vi "SOUR_POW_CORR_COLL_ITER_NTOL.vi"(0 "VISA IN":refnum<visa-resource-name>, 1 "Port number":i32, 2 "Tolerance Value(dBm)":dbl, 5 "error in":errorcluster, 7 "Channel":i32) -> (14 "VISA Out":refnum<visa-resource-name>, 19 "error out":errorcluster)   [LabVIEW 2018, in "PNA-X.lvlib"]
doc: "SOURce:POWer:CORRection:COLLect:ITERation:NTOLerance <num> \n1839\n\n(Read-Write) This command, along with SOUR:POW:CORR:COLL:ITER:COUNT describes the \nnumber of ADUSTMENTS to make to the source power. \nSets the maximum desired deviation from the sum of the test port power and the offset value. Power \nREADINGS (performed by SOUR:POW:CORR:COLL:AVER:COUNT and \nSOUR:POW:CORR:COLL:AVER:NTOLerance) will continue to be made, and source power \nadjusted, until a measurement is within this tolerance value or the max number of measurements has \nbeen met. The last value is the valid measurement for that data point. \nLearn more. \nParameters \n<cnum> Any existing channel number. If unspecified, value is set to 1 \n<port> Port number to correct for source power. If unspecified, value is set to 1. \n<num> Tolerance value in dBm. Choose any number between 0 and 5 \nExamples SOUR:POW:CORR:COLL:ITER:NTOL .005 \nsource:power:correction:collect:iteration:ntolerance .1 \nQuery Syntax SOURce:POWer:CORRection:COLLect:ITERation:NTOLerance? \nReturn Type Numeric \nDefault .05 \nSOURce<cnum>:POWer<port>:CORRection:COLLect:METHod <char> Superseded \nThis command is replaced with SOUR:POW:CORR:COLLect[:ACQuire] which now specifies the \nmethod and the device. \n(Read-Write) Selects the calibration method to be used for the source power cal acquisition. \nParameters \n<cnum> Any existing channel number. If unspecified, value is set to 1 \n<port> Port number to correct for source power. If unspecified, value is set to 1. \n<char> Choose from: \nNONE - No Cal method \nPMETer - Power Meter is used for all readings. (same as \"fast iteration\" box \nnot checked on dialog box) \nPMReceiver - Power meter for the first iteration; then use the reference \nreceiver for remaining readings if necessary (same as \"fast iteration\" box \n1840\n\nchecked on dialog box) \nExamples SOUR:POW:CORR:COLL:METH PMET \nsource1:power2:correction:collect:method pmreceiver \nQuery Syntax SOURce:POWer:CORRection:COLLect:METHod? \nReturn Type Character \nDefault NONE \nSOURce<cnum>:POWer<port>:CORRection:COLLect:SAVE [<RREC>] \n(Write-only) Applies the array of correction values after a source power calibration sweep has \ncompleted. The source power correction will then be active on the specified source port for channel \n<cnum>. This command does NOT save the correction values. To save correction values, save an \ninstrument / calibration state (*.cst file) after performing a source power cal. \nParameters \n<cnum> Any existing channel number. If unspecified, value is set to 1 \n<port> Port number to correct for source power. If unspecified, value is set to 1. \n<RREC> Optional argument. \nRRECeiver In addition to a source Power Cal, perform a calibration of the \nreference receiver used in the measurement. ONLY the Reference Receiver \ncalibration is then saved to a Cal Set or Cal Register as specified by the current \nsetting of SENS:CORR:PREF:CSET:SAVE. \nExamples SOUR:POW:CORR:COLL:SAVE \nsource1:power2:correction:collect:save rreceiver \nQuery Syntax Not Applicable \nDefault Not Applicable \nSOURce<cnum>:POWer:CORRection:COLLect:<pmChan>SENsor[:FRANge] \n<num1>,<num2> \n1841\n\n(Read-Write) Specifies the frequency range over which the power sensors connected to the specified \nchannels (A and B) of the power meter can be used (minimum frequency, maximum frequency). If the \npower meter has only a single channel, that channel is considered channel A. \nParameters \n<cnum> Any existing channel number. If unspecified, value is set to 1 \n<pmChan> Power Meter channel. Choose from: \nA - Channel A \nB - Channel B \n<num1> Minimum frequency for the sensor. If a frequency unit is not specified, Hz is \nassumed. No limits are placed on this value. \n<num2> Maximum frequency for the sensor. If a frequency unit is not specified, Hz is \nassumed. No limits are placed on this value. \nExamples SOUR:POW:CORR:COLL:ASEN 100E3, 3E9 \nsource1:power2:correction:collect:bsensor:frange 10 MHz, 18 GHz \nQuery Syntax SOURce:POWer:CORRection:COLLect:ASENsor[:FRANge]?"
uses:
  PNA-X.lvlib
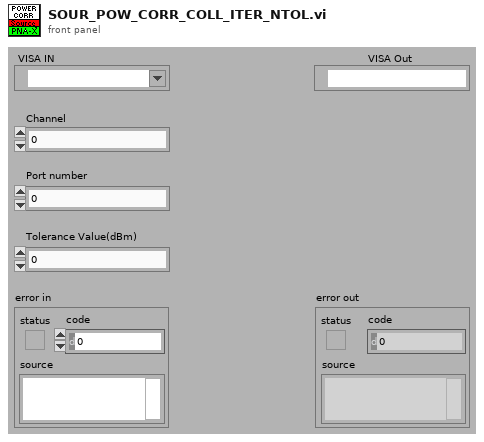
[diagram p1: front panel]
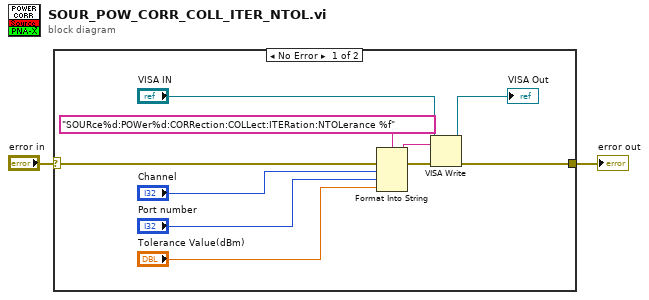
[diagram p0: block diagram]
diagram:
  n1 = case shown="No Error" "error in" {
    selector: "error in" -> [w12 w13]
    tunnel: [w7 w13] -> w1
    frame No Error {
      n2 = Format Into String(format string="SOURce%d:POWer%d:CORRection:COLLect:ITERation:NTOLerance %f" ("Cmdline"), error in=w12, "Channel", "Port number", "Tolerance Value(dBm)") -> (resulting string=w10:string, error out=w11:errorcluster)  [unwired: 1 in]
      n3 = VISA Write(VISA resource name="VISA IN", write buffer=w10, error in (no error)=w11) -> (VISA resource name out=→"VISA Out":refnum<visa-resource-name>, error out=w7:errorcluster)  [unwired: 1 out]
    }
    frame Error {
    }
  }
  "error out" <- w1
